vi "CRYPIC PUSH Message to MainMenu.vi"(9 "cMsgProject":T1) -> ()   [LabVIEW 2013]
uses:
  CRYMain Sub Window Global.vi
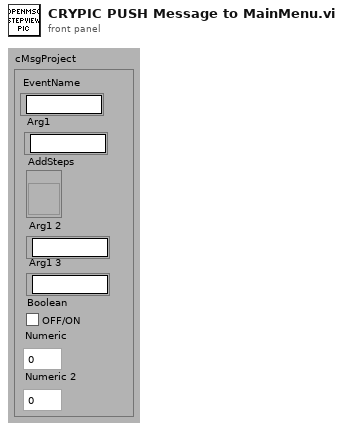
[diagram p1: front panel]
types:
  T1 = cluster{"EventName":string, "Arg1":string, "Numeric":u16, "Numeric 2":u16, "AddSteps ":refnum<vi>, "Arg1 2":string, "Arg1 3":string, "Boolean":bool}
  T2 = cluster{"cMsgProjectList":cluster{"EventName":string, "Arg1":string, "Numeric":u16, "Numeric 2":u16, "AddSteps ":refnum<vi>, "Arg1 2":string, "Arg1 3":string, "Boolean":bool}[], "nIDList":i32[]}
  T3 = cluster{"EventName":string, "Arg1":string, "Numeric":u16, "Numeric 2":u16, "AddSteps ":refnum<vi>, "Arg1 2":string, "Arg1 3":string, "Boolean":bool}[]
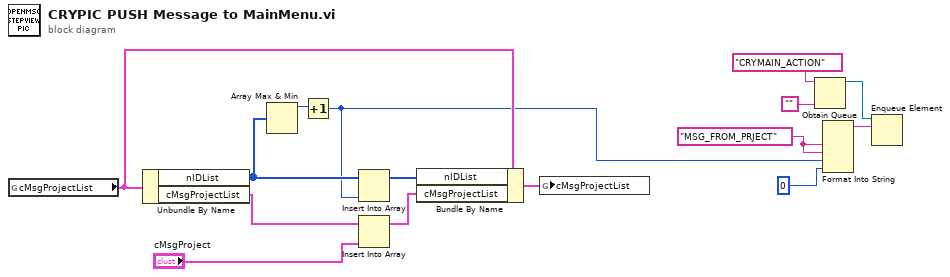
[diagram p0: block diagram]
diagram:
  w10 = "MSG_FROM_PRJECT" ("input 1")
  n1 = global read "CRYMain Sub Window Global.vi" "cMsgProjectList"() -> (w5:T2)
  n2 = Unbundle By Name(w5) -> ("nIDList"=w8:i32[], "cMsgProjectList"=w7:T3)
  n3 = Array Max & Min(array=w8) -> (max value=w9:i32)  [unwired: 3 out]
  n4 = Increment(x=w9) -> (x+1=w1:i32)
  n5 = Insert Into Array(array=w8, new element=w1) -> (w4:i32[])  [unwired: 1 in]
  n6 = Insert Into Array(array=w7, new element="cMsgProject") -> (w3:T3)  [unwired: 1 in]
  n7 = Bundle By Name(cluster=w5, "nIDList"=w4, "cMsgProjectList"=w3) -> (w2:T2)
  n8 = global write "CRYMain Sub Window Global.vi" "cMsgProjectList"(w2) -> ()
  n9 = Obtain Queue(name (unnamed)="CRYMAIN_ACTION" ("YAxisTitle"), element data type="" ("Action Type")) -> (queue out=w12:refnum<queue>)  [unwired: 3 in, 2 out]
  n10 = Format Into String(w10, w10, w1, 0 ("input 3")) -> (resulting string=w13:string)  [unwired: 3 in, 1 out]
  n11 = Enqueue Element(queue=w12, element=w13) -> ()  [unwired: 1 in, 4 out]
